vi "Camera_ID.vi"(8 "error in":errorcluster, 11 "CAM_ID":T1) -> (0 "error out":errorcluster, 1 "CAM2":string, 2 "CAM1":string, 3 "CAM_ID out":T1)   [LabVIEW 2022 SP3]
uses:
  CAM_ID.ctl
  <vilib>/vision/driver/NI_Vision_Acquisition_Software.lvlib
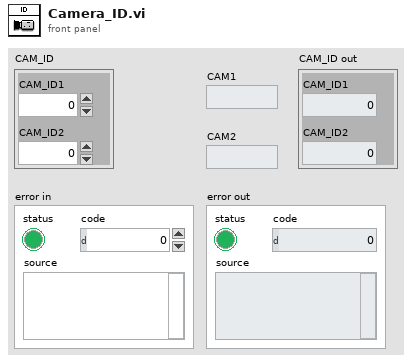
[diagram p1: front panel]
types:
  T1 = typedef "CAM_ID.ctl" = cluster{"CAM_ID1":i32, "CAM_ID2":i32}
  T2 = cluster{"Type":u32, "Version":u32, "Flags":u32, "SerialNumberHigh":u32, "SerialNumberLow":u32, "BusType":u32, "InterfaceName":string, "VendorName":string, "ModelName":string, "CameraFileName":string, "CameraAttributeURL":string}[]
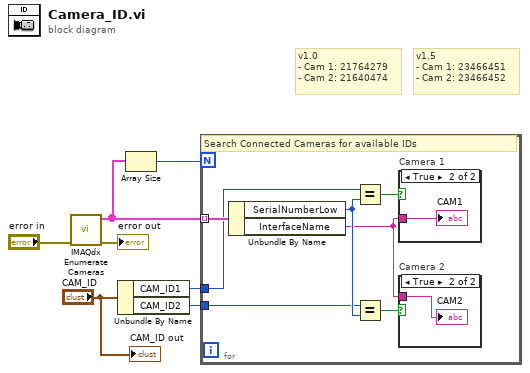
[diagram p0: block diagram]
diagram:
  # "v1.5\n- Cam 1: 23466451 \n- Cam 2: 23466452"
  # "v1.0\n- Cam 1: 21764279 \n- Cam 2: 21640474"
  n1 = call <vilib>:"IMAQdx Enumerate Cameras.vi"("error in"="error in") -> ("error out"=→"error out":errorcluster, "Camera Information Array"=w6:T2)  [unwired: 9 in]
  n2 = Unbundle By Name("CAM_ID") -> ("CAM_ID1"=w2:i32, "CAM_ID2"=w1:i32)
  n3 = Array Size(array=w6) -> (size(s)=w7:i32)
  n4 = for {
    N: w7 -> [_]
    tunnel: w6 -> [w14] mode=indexing
    tunnel: w2 -> [w13]
    tunnel: w1 -> [w11]
    # "Search Connected Cameras for available IDs"
    n5 = Unbundle By Name(w14) -> ("SerialNumberLow"=w12:u32, "InterfaceName"=w8:string)
    n6 = Equal?(x=w13, y=w12) -> (x = y?=w10:bool)
    n7 = Equal?(x=w11, y=w12) -> (x = y?=w9:bool)
    n8 = case "Camera 1" shown="True" w10 {
      tunnel: w8 -> [_ w16]
      frame False {
      }
      frame True {
        "CAM1" <- w16
      }
    }
    n9 = case "Camera 2" shown="True" w9 {
      tunnel: w8 -> [_ w15]
      frame False {
      }
      frame True {
        "CAM2" <- w15
      }
    }
  }
  "CAM_ID out" <- "CAM_ID"
